vi "Query Window (serial).vi"() -> ()   [LabVIEW 2011]
uses:
  <vilib>/Instr/_visa.llb/VISA Configure Serial Port (Instr).vi
panel:
  in  "Query":bool
  in  "VISA resource name 2":refnum<visa-resource-name>
  out "read buffer":string
  in  "write buffer":string
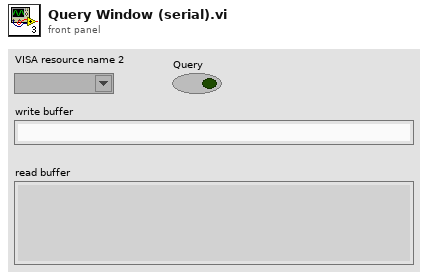
[diagram p1: front panel]
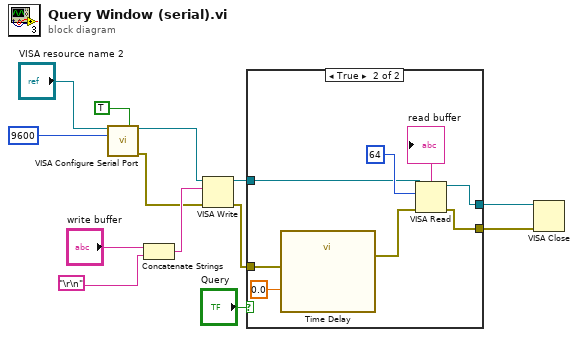
[diagram p0: block diagram]
diagram:
  n1 = call-poly "VISA Configure Serial Port"("VISA resource name"="VISA resource name 2", "Enable Termination\nChar (T)"=TRUE ("Enable Termination\nChar (T)"), "baud rate (9600)"=u32 9600) -> ("VISA resource name out"=w6:refnum<visa-resource-name>, "error out"=w7:errorcluster)  [unwired: 11 in]
  n2 = Concatenate Strings("write buffer", "\r\n") -> (w11:string)
  n3 = VISA Write(VISA resource name=w6, write buffer=w11, error in (no error)=w7) -> (VISA resource name out=w13:refnum<visa-resource-name>, error out=w4:errorcluster)  [unwired: 1 out]
  n4 = case shown="True" "Query" {
    tunnel: w13 -> [w15 w21]
    tunnel: w4 -> [w14 w20]
    tunnel: [w14 w17] -> w3
    tunnel: [w15 w16] -> w2
    frame False {
    }
    frame True {
      n5 = call "Time Delay"("error in (no error)"=w20, "Delay Time (s)"=0.0) -> ("error out"=w19:errorcluster)  [unwired: 9 in]
      n6 = VISA Read(VISA resource name=w21, byte count=u32 64, error in (no error)=w19) -> (VISA resource name out=w16:refnum<visa-resource-name>, read buffer=→"read buffer":string, error out=w17:errorcluster)  [unwired: 1 out]
    }
  }
  n7 = VISA Close(VISA resource name=w2, error in (no error)=w3) -> ()  [unwired: 1 out]
